vi "Main.vi"() -> ()   [LabVIEW 2022 SP3]
panel:
  out "Day 1 Part 2":u32
  out "Day 1 Part 1":u32
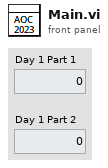
[diagram p1: front panel]
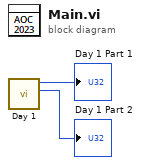
[diagram p0: block diagram]
diagram:
  n1 = call "Day 1.vi"() -> ("Part 2"=→"Day 1 Part 2":u32, "Part 1"=→"Day 1 Part 1":u32)  [unwired: 9 in, 1 out]
